vi "Day 4 - Ceres Search.vi"() -> ()   [LabVIEW 2020, in "AoC 2024.lvlib"]
uses:
  AoC 2024.lvlib
  249bf285-18d4-446a-9567-11d62d8269c1.vi
  49e0b310-a5fb-4790-b923-753cda70fba4.vi
  <userlib>/_OpenG.lib/string/string.llb/openg_string.lvlib
panel:
  out "Puzzle Part-2 Answer":string
  out "Puzzle Answer":string
  in  "Puzzle Input":string="MMMSXXMASM\nMSAMXMSMSA\nAMXSXMAAMM\nMSAMASMSMX\nXMASAMXAMM\nXXAMMXXAMA\nSMSMSASXSS\nSAXAMASAAA\nMAMMMXMMMM\nMXMXAXMASX"
  # "Enter the Puzzle Input and run the VI"
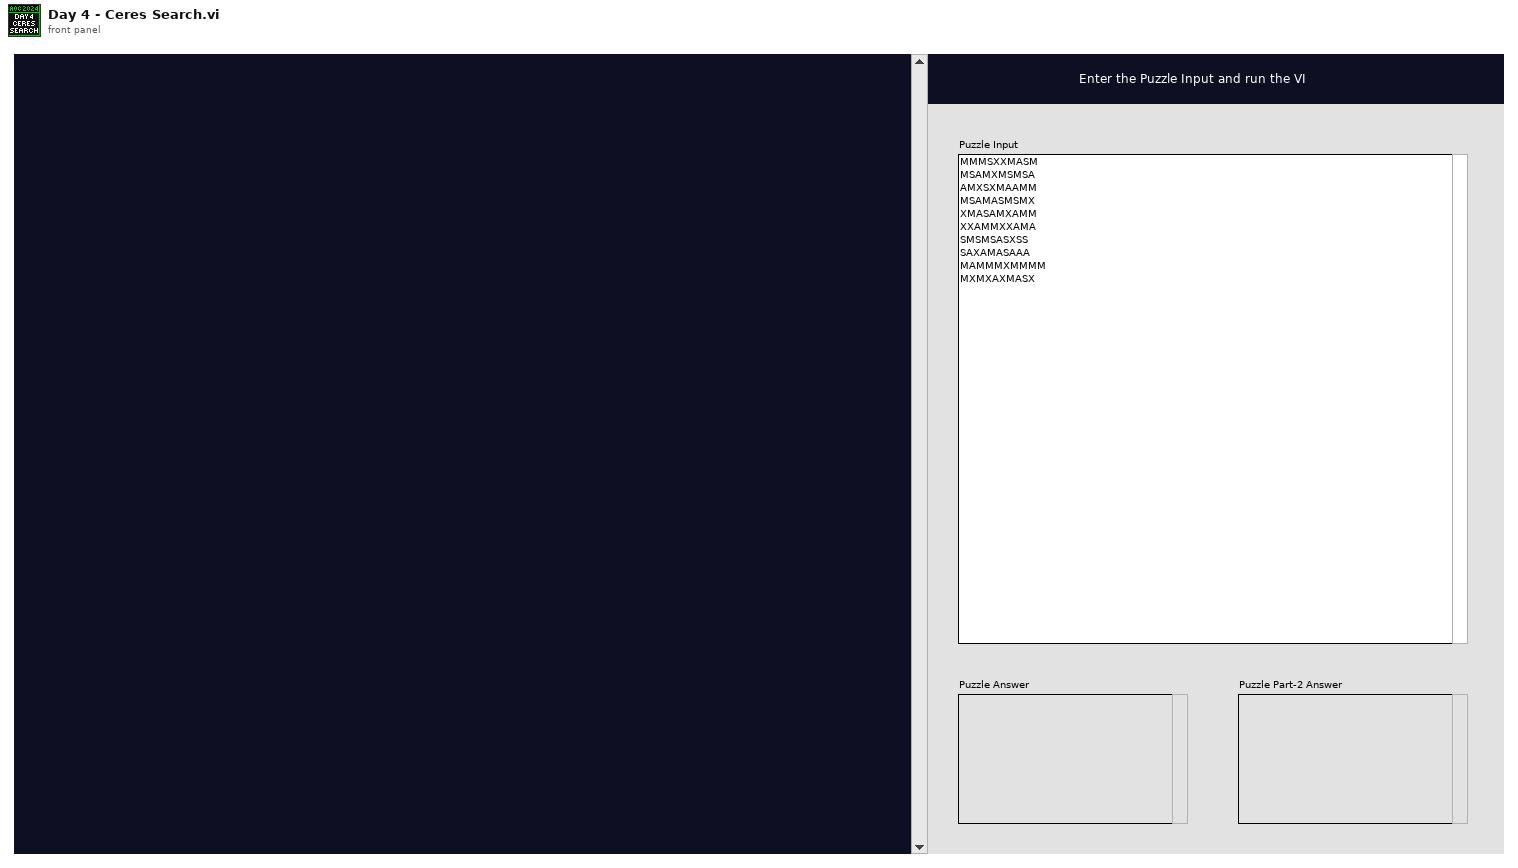
[diagram p1: front panel]
types:
  T1 = enum16{"Left", "Right", "Up", "Down", "Left Up", "Left Down", "Right Up", "Right Down"}
  T2 = enum16{"Left", "Right", "Up", "Down", "Left Up", "Left Down", "Right Up", "Right Down"}[]
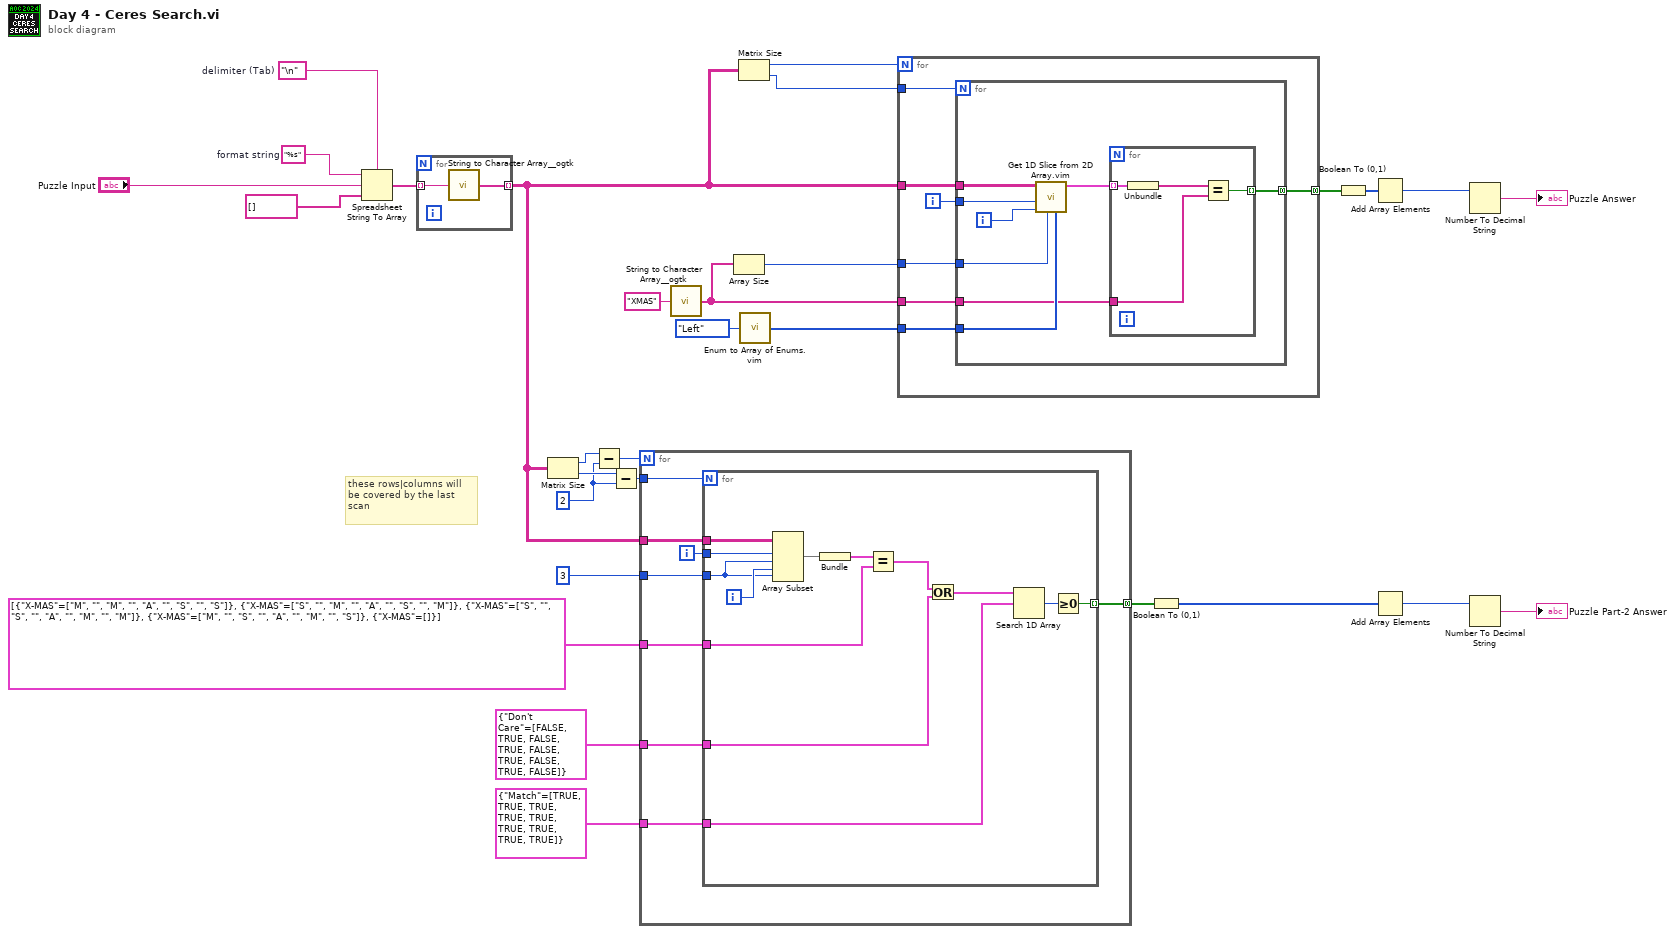
[diagram p0: block diagram]
diagram:
  w1 = 2 ("y")
  w26 = "\n"  # delimiter (Tab)
  w27 = "%s"  # format string
  # "these rows|columns will be covered by the last scan"
  n1 = Spreadsheet String To Array(delimiter (Tab)=w26, format string=w27, spreadsheet string="Puzzle Input", array type (2D Dbl)=string[] []) -> (array=w24:string[])
  n2 = for {
    tunnel: w24 -> [w31] mode=indexing
    tunnel: [w32] -> w13 mode=indexing
    n3 = call <userlib>:"String to Character Array__ogtk.vi"("Input String"=w31) -> ("Character Array"=w32:string[])
  }
  n4 = Matrix Size(0:w13) -> (1:w12:i32, 2:w11:i32)
  n5 = Subtract(x=w12, y=w1) -> (x-y=w10:i32)
  n6 = Subtract(x=w11, y=w1) -> (x-y=w9:i32)
  n7 = for {
    N: w10 -> [_]
    tunnel: w13 -> [w39]
    tunnel: w9 -> [w40]
    tunnel: 3 ("y") -> [w37]
    tunnel: cluster{"X-MAS":string[][]}[] [{"X-MAS"=[["M", "", "M"], ["", "A", ""], ["S", "", "S"]]}, {"X-MAS"=[["S", "", "M"], ["", "A", ""], ["S", "", "M"]]}, {"X-MAS"=[["S", "", "S"], ["", "A", ""], ["M", "", "M"]]}, {"X-MAS"=[["M", "", "S"], ["", "A", ""], ["M", "", "S"]]}, {"X-MAS"=[]}] -> [w36]
    tunnel: cluster{"Don't Care":bool[][]} {"Don't Care"=[[FALSE, TRUE, FALSE], [TRUE, FALSE, TRUE], [FALSE, TRUE, FALSE]]} -> [w35]
    tunnel: cluster{"Match":bool[][]} {"Match"=[[TRUE, TRUE, TRUE], [TRUE, TRUE, TRUE], [TRUE, TRUE, TRUE]]} -> [w34]
    tunnel: [w33] -> w5 mode=concatenating
    i -> [w38]
    n8 = for {
      N: w40 -> [_]
      tunnel: w39 -> [w53]
      tunnel: w38 -> [w52]
      tunnel: w37 -> [w50]
      tunnel: w36 -> [w47]
      tunnel: w35 -> [w45]
      tunnel: w34 -> [w43]
      tunnel: [w41] -> w33 mode=indexing
      i -> [w51]
      n9 = Array Subset(array=w53, index (row)=w52, length (row)=w50, index (col)=w51, length (col)=w50) -> (w49:string[][])
      n10 = Bundle(w49) -> (w48:cluster{string[][]})  [unwired: 1 in]
      n11 = Equal?(x=w48, y=w47) -> (x = y?=w46:cluster{bool[][]}[])
      n12 = Or(x=w46, y=w45) -> (x .or. y?=w44:cluster{bool[][]}[])
      n13 = Search 1D Array(1D array=w44, element=w43) -> (index of element=w42:i32)  [unwired: 1 in]
      n14 = Greater Or Equal To 0?(x=w42) -> (x >= 0?=w41:bool)
    }
  }
  n15 = call <userlib>:"String to Character Array__ogtk.vi"("Input String"="XMAS") -> ("Character Array"=w18:string[])
  n16 = Array Size(array=w18) -> (size(s)=w14:i32)
  n17 = Matrix Size(0:w13) -> (1:w23:i32, 2:w22:i32)
  n18 = call "Enum to Array of Enums.vim"("enum"=T1."Left" ("Direction")) -> ("array of enums"=w19:T2)
  n19 = for {
    N: w23 -> [_]
    tunnel: w13 -> [w59]
    tunnel: w22 -> [w60]
    tunnel: w14 -> [w57]
    tunnel: w19 -> [w56]
    tunnel: w18 -> [w55]
    tunnel: [w54] -> w16 mode=concatenating
    i -> [w58]
    n20 = for {
      N: w60 -> [_]
      tunnel: w59 -> [w68]
      tunnel: w58 -> [w66]
      tunnel: w57 -> [w67]
      tunnel: w56 -> [w64]
      tunnel: w55 -> [w63]
      tunnel: [w61] -> w54 mode=concatenating
      i -> [w65]
      n21 = call "Get 1D Slice from 2D Array.vim"("Direction"=w64, "length"=w67, "index (col)"=w65, "index (row)"=w66, "2D Array"=w68) -> ("1D Slice"=w62:cluster{string[]}[])  [unwired: 4 in]
      n22 = for {
        tunnel: w63 -> [w70]
        tunnel: w62 -> [w72] mode=indexing
        tunnel: [w69] -> w61 mode=indexing
        n23 = Unbundle(w72) -> (w71:string[])
        n24 = Equal?(x=w71, y=w70) -> (x = y?=w69:bool)
      }
    }
  }
  n25 = Boolean To (0,1)(Boolean=w5) -> (0, 1=w4:i16[])
  n26 = Boolean To (0,1)(Boolean=w16) -> (0, 1=w17:i16[])
  n27 = Add Array Elements(numeric array=w17) -> (sum=w15:i16)
  n28 = Add Array Elements(numeric array=w4) -> (sum=w3:i16)
  n29 = Number To Decimal String(number=w15) -> (decimal integer string=→"Puzzle Answer":string)  [unwired: 1 in]
  n30 = Number To Decimal String(number=w3) -> (decimal integer string=→"Puzzle Part-2 Answer":string)  [unwired: 1 in]
